vi "Prog4.vi"() -> ()   [LabVIEW 2021]
panel:
  out "length 3":i32
  out "length 2":i32
  out "length":i32
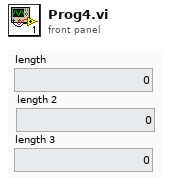
[diagram p1: front panel]
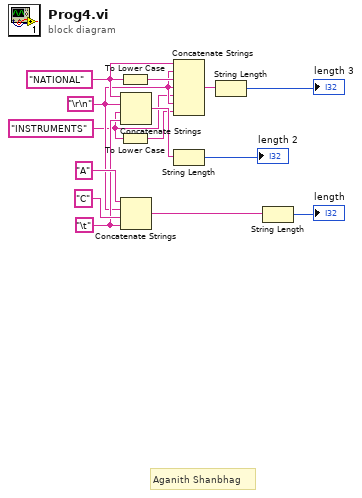
[diagram p0: block diagram]
diagram:
  w10 = "\t"
  w5 = "\r\n"
  w3 = "INSTRUMENTS"
  w7 = "NATIONAL"
  # "Aganith Shanbhag"
  n1 = To Lower Case(string=w7) -> (all lower case string=w6:string)
  n2 = To Lower Case(string=w3) -> (all lower case string=w4:string)
  n3 = Concatenate Strings(w7, w5, w3, w10) -> (w9:string)
  n4 = Concatenate Strings "Concatenate Strings"("A", w5, "C", w10) -> (w12:string)
  n5 = Concatenate Strings(w7, w5, w6, w5, w3, w5, w4) -> (w1:string)
  n6 = String Length(string=w9) -> (length=→"length 2":i32)
  n7 = String Length(string=w1) -> (length=→"length 3":i32)
  n8 = String Length(string=w12) -> (length=→"length":i32)
